vi "fourier_ring_correlation.vi"(9 "img2":dbl[][](array[numeric]), 10 "img1":dbl[][](array[numeric])) -> (1 "frc mean":dbl format="%0.2f", 2 "frc curve":dbl[][](graph))   [LabVIEW 2017]
uses:
  <vilib>/Analysis/2dsp.llb/2D Real FFT.vi
  <vilib>/Analysis/baseanly.llb/Mean (DBL).vi
  <vilib>/Analysis/3filter.llb/Zero Phase Filter (DBL).vi
  <vilib>/Analysis/NI_AALPro.lvlib
  <vilib>/Analysis/NI_AALBase.lvlib
panel:
  in  "debug":bool
  in  "power":dbl=0.1 format="%#_13g"
  out "Image":T1(plugin-control)
  in  "File Path 2":path=path "C:/Users/SiMView/Pictures/idle state-1.tif"
  in  "File Path":path=path "C:/Users/SiMView/Pictures/idle state.tif"
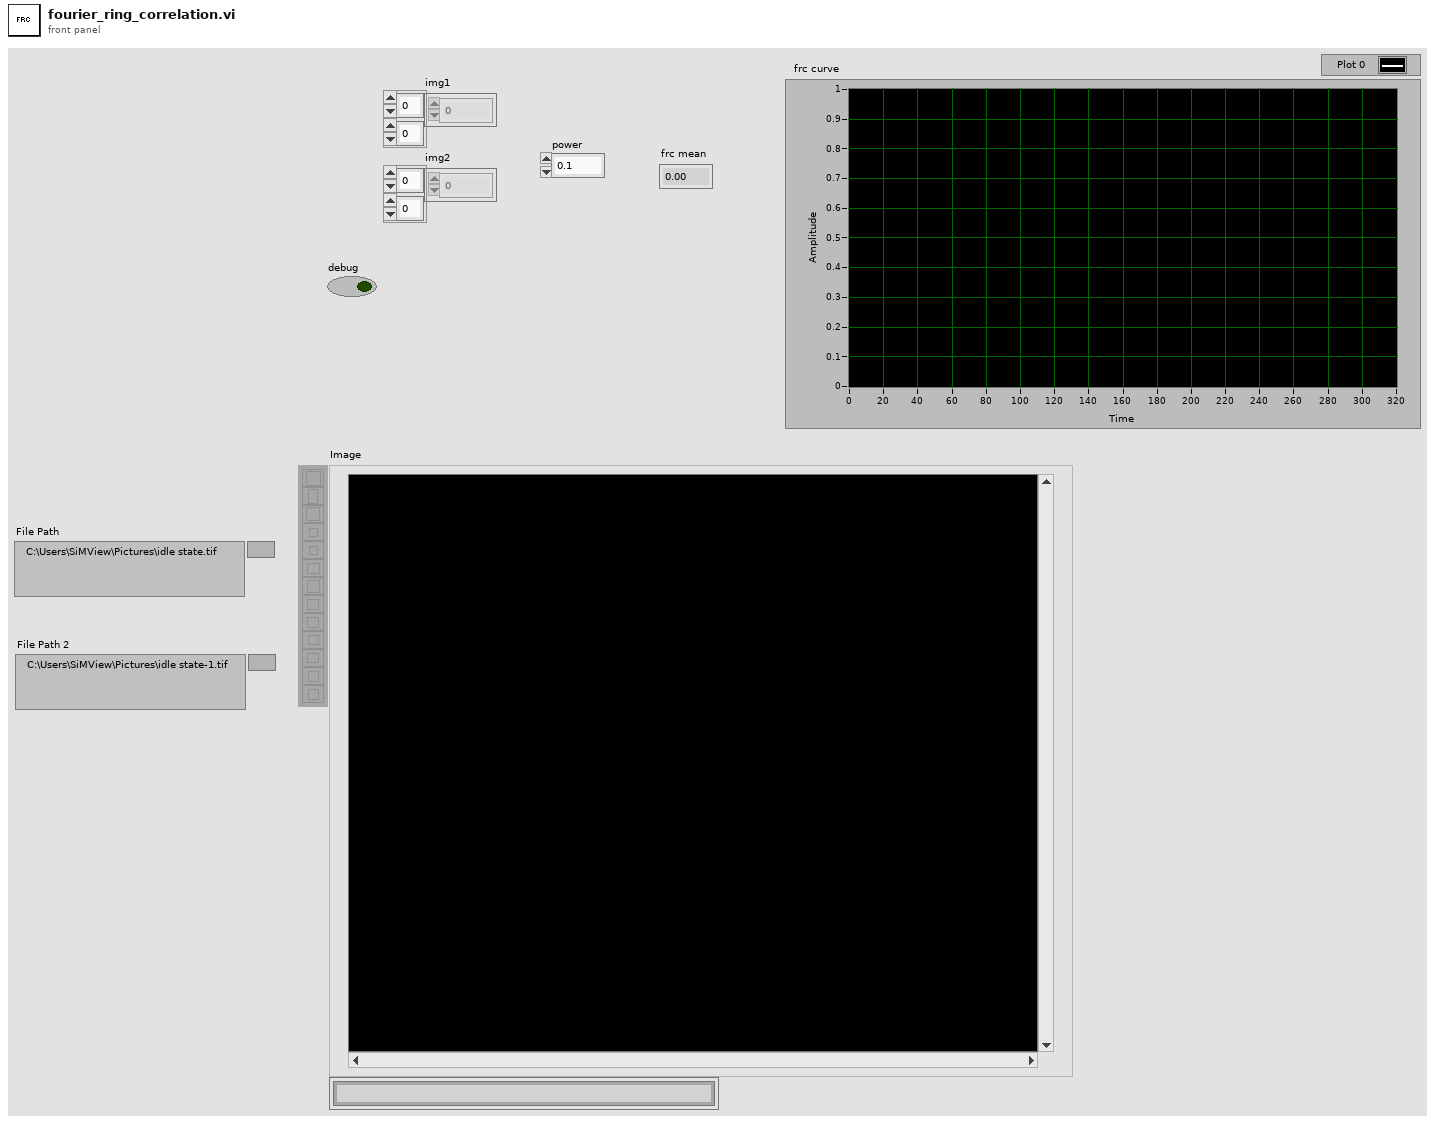
[diagram p1: front panel]
types:
  T1 = typedef "IMAQ Image.ctl" = refnum<image>
  T2 = typedef "Image Type" = u32
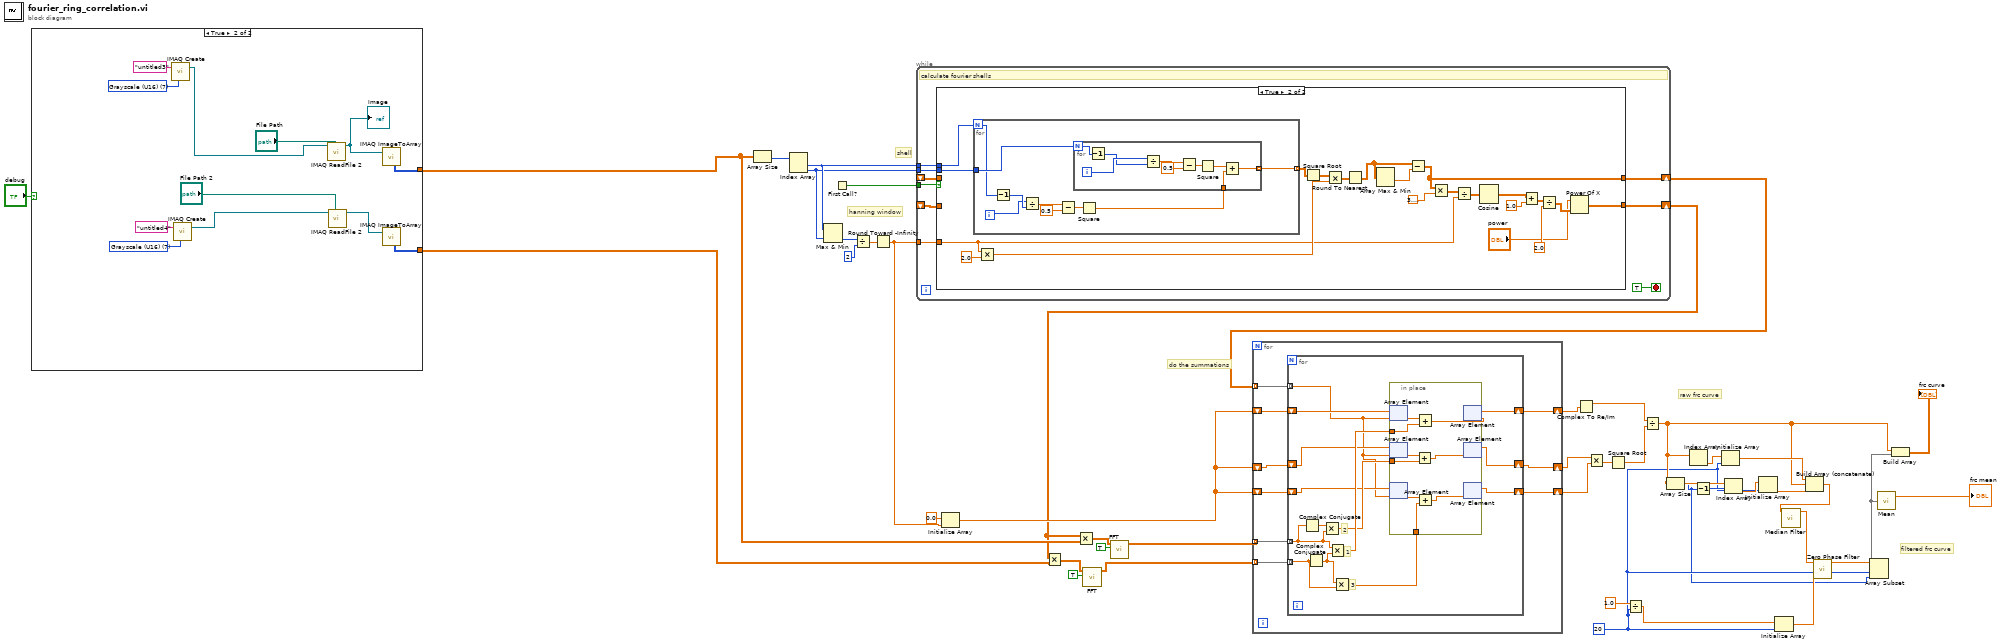
[diagram p0: block diagram]
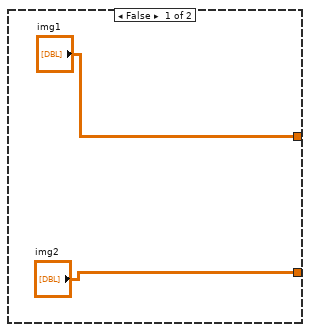
[diagram p2: hidden frame]
diagram:
  w14 = 20 ("dimension size")
  # "filtered frc curve"
  # "raw frc curve"
  # "do the summations"
  # "hanning window"
  # "shell"
  n1 = case shown="True" "debug" {
    tunnel: ["img1" w49] -> w5
    tunnel: ["img2" w47] -> w4
    frame False {
    }
    frame True {
      w53 = T2 7 items=["Grayscale (U8)", "Grayscale (I16)", "Grayscale (SGL)", "Complex (CSG)", "RGB (U32)", "HSL (U32)", "RGB (U64)", "Grayscale (U16)"] ("Image Type")
      w55 = T2 7 items=["Grayscale (U8)", "Grayscale (I16)", "Grayscale (SGL)", "Complex (CSG)", "RGB (U32)", "HSL (U32)", "RGB (U64)", "Grayscale (U16)"] ("Image Type")
      n2 = call "IMAQ Create"("Image Name"="untitled3", "Image Type"=w55) -> ("New Image"=w54:T1)  [unwired: 3 in, 1 out]
      n3 = call "IMAQ Create"("Image Name"="untitled4", "Image Type"=w53) -> ("New Image"=w51:T1)  [unwired: 3 in, 1 out]
      n4 = call "IMAQ ReadFile 2"("File Path"="File Path", "Image"=w54) -> ("Image Out"=w50:T1)  [unwired: 5 in, 4 out]
      "Image" <- w50
      n5 = call "IMAQ ReadFile 2"("File Path"="File Path 2", "Image"=w51) -> ("Image Out"=w48:T1)  [unwired: 5 in, 4 out]
      n6 = call "IMAQ ImageToArray"("Image"=w50) -> ("Image Pixels (U16)"=w49:u16[][])  [unwired: 3 in, 4 out]
      n7 = call "IMAQ ImageToArray"("Image"=w48) -> ("Image Pixels (U16)"=w47:u16[][])  [unwired: 3 in, 4 out]
    }
  }
  n8 = Array Size(array=w5) -> (size(s)=w44:i32[])
  n9 = Index Array(array=w44) -> (element #1=w40:i32, element #2=w39:i32)  [unwired: 2 in]
  n10 = Max & Min(x=w40, y=w39) -> (min(x,y)=w41:i32)  [unwired: 1 out]
  n11 = First Call?() -> (First Call?: T/F=w10:bool)
  n12 = Divide(x=w41, y=2) -> (x/y=w42:dbl)
  n13 = Round Toward -Infinity(1:w42) -> (0:w37:dbl)
  n14 = while {
    tunnel: w40 -> [w67]
    tunnel: w39 -> [w66]
    tunnel: w37 -> [w65]
    tunnel: w10 -> [w64]
    shift-right: [w61] -> w3
    shift-left: _ -> [w62]
    shift-right: [w59] -> w2
    shift-left: _ -> [w60]
    stop <- TRUE stop-if-true
    # "calculate fourier shells"
    n15 = case shown="True" w64 {
      tunnel: w67 -> [_ w90]
      tunnel: w66 -> [_ w89]
      tunnel: w65 -> [_ w78]
      tunnel: w62 -> [w69 _]
      tunnel: [w69 w81] -> w61
      tunnel: w60 -> [w68 _]
      tunnel: [w68 w72] -> w59
      frame False {
      }
      frame True {
        n16 = for {
          N: w90 -> [w95]
          tunnel: w89 -> [w99]
          tunnel: [w91] -> w86 mode=indexing
          i -> [w94]
          n17 = Decrement(x=w95) -> (x-1=w96:i32)
          n18 = Divide(x=w94, y=w96) -> (x/y=w97:dbl)
          n19 = Subtract(x=w97, y=0.5) -> (x-y=w93:dbl)
          n20 = Square(x=w93) -> (x^2=w92:dbl)
          n21 = for {
            N: w99 -> [w107]
            tunnel: w92 -> [w101]
            tunnel: [w100] -> w91 mode=indexing
            i -> [w108]
            n22 = Decrement(x=w107) -> (x-1=w106:i32)
            n23 = Divide(x=w108, y=w106) -> (x/y=w105:dbl)
            n24 = Subtract(x=w105, y=0.5) -> (x-y=w103:dbl)
            n25 = Square(x=w103) -> (x^2=w102:dbl)
            n26 = Add(x=w102, y=w101) -> (x+y=w100:dbl)
          }
        }
        n27 = Multiply(x=w78, y=2.0) -> (x*y=w84:dbl)
        n28 = Square Root(x=w86) -> (sqrt(x)=w87:dbl[][])
        n29 = Multiply(x=w87, y=w84) -> (x*y=w88:dbl[][])
        n30 = Round To Nearest(number=w88) -> (nearest integer value=w82:dbl[][])
        n31 = Array Max & Min(array=w82) -> (min value=w83:dbl)  [unwired: 3 out]
        n32 = Subtract(x=w82, y=w83) -> (x-y=w81:dbl[][])
        n33 = Multiply(x=w81, y=3.141592653589793) -> (x*y=w79:dbl[][])
        n34 = Divide(x=w79, y=w78) -> (x/y=w77:dbl[][])
        n35 = Cosine(x=w77) -> (cos(x)=w76:dbl[][])
        n36 = Add(x=w76, y=1.0) -> (x+y=w74:dbl[][])
        n37 = Divide(x=w74, y=2.0) -> (x/y=w71:dbl[][])
        n38 = Power Of X(1:w71, 2:"power") -> (0:w72:dbl[][])
      }
    }
  }
  n39 = Initialize Array(0.0 ("element"), w37) -> (w36:dbl[])
  n40 = Multiply(x=w2, y=w4) -> (x*y=w9:dbl[][])
  n41 = Multiply(x=w2, y=w5) -> (x*y=w7:dbl[][])
  n42 = call-poly <vilib>:"FFT.vi"("shift?"=TRUE, "X"=w9) -> ("FFT {X}"=w8:cdb[][])  [unwired: 8 in, 1 out]
  n43 = call-poly <vilib>:"FFT.vi"("shift?"=TRUE, "X"=w7) -> ("FFT {X}"=w6:cdb[][])  [unwired: 8 in, 1 out]
  n44 = for {
    tunnel: w6 -> [w111] mode=indexing
    tunnel: w8 -> [w110] mode=indexing
    tunnel: w3 -> [w109] mode=indexing
    shift-right: [w114] -> w32
    shift-left: w36 -> [w117]
    shift-right: [w113] -> w35
    shift-left: w36 -> [w116]
    shift-right: [w112] -> w34
    shift-left: w36 -> [w115]
    n45 = for {
      tunnel: w109 -> [w120] mode=indexing
      tunnel: w111 -> [w130] mode=indexing
      tunnel: w110 -> [w128] mode=indexing
      shift-right: [w125] -> w114
      shift-left: w117 -> [w127]
      shift-right: [w122] -> w113
      shift-left: w116 -> [w124]
      shift-right: [w118] -> w112
      shift-left: w115 -> [w121]
      # "3"
      # "2"
      # "1"
      n46 = Complex Conjugate(1:w130) -> (0:w131:cdb)
      n47 = Complex Conjugate(1:w128) -> (0:w129:cdb)
      n48 = Multiply(x=w131, y=w130) -> (x*y=w123:cdb)
      n49 = Multiply(x=w130, y=w129) -> (x*y=w126:cdb)
      n50 = Multiply(x=w129, y=w128) -> (x*y=w119:cdb)
      n51 = in-place {
        in-place-border: w126 -> [w139]
        in-place-border: w123 -> [w136]
        in-place-border: w119 -> [w133]
        n52 = in-place-array #1(w127, w120) -> (w140:dbl)
        n53 = in-place-array #2(w124, w120) -> (w137:dbl)
        n54 = in-place-array #3(w121, w120) -> (w134:dbl)
        n55 = Add(x=w137, y=w136) -> (x+y=w135:cdb)
        n56 = Add(x=w140, y=w139) -> (x+y=w138:cdb)
        n57 = Add(x=w134, y=w133) -> (x+y=w132:cdb)
        n58 = in-place-array #1(w138) -> (w125:dbl[])  [unwired: 1 out]
        n59 = in-place-array #2(w135) -> (w122:dbl[])  [unwired: 1 out]
        n60 = in-place-array #3(w132) -> (w118:dbl[])  [unwired: 1 out]
      }
    }
  }
  n61 = Complex To Re/Im(x + iy=w32) -> (x=w31:dbl[])  [unwired: 1 out]
  n62 = Multiply(x=w35, y=w34) -> (x*y=w33:dbl[])
  n63 = Square Root(x=w33) -> (sqrt(x)=w30:dbl[])
  n64 = Divide(x=1.0 ("element"), y=w14) -> (x/y=w23:dbl)
  n65 = Divide(x=w31, y=w30) -> (x/y=w19:dbl[])
  n66 = Array Size(array=w19) -> (size(s)=w13:i32)
  n67 = Index Array(array=w19) -> (element=w22:dbl)  [unwired: 1 in]
  n68 = Decrement(x=w13) -> (x-1=w20:i32)
  n69 = Initialize Array(w22, w14) -> (w21:dbl[])
  n70 = Index Array(array=w19, index=w20) -> (element=w18:dbl)
  n71 = Initialize Array(w18, w14) -> (w17:dbl[])
  n72 = Initialize Array(w23, w14) -> (w27:dbl[])
  n73 = Build Array (concatenate)(w21, w19, w17) -> (w16:dbl[])
  n74 = call <vilib>:"Median Filter.vi"("X"=w16) -> ("Filtered X"=w25:dbl[])  [unwired: 9 in, 1 out]
  n75 = call-poly <vilib>:"Zero Phase Filter.vi"("Forward Coefficients"=w27, "X"=w25) -> ("Filtered X"=w15:dbl[])  [unwired: 8 in, 1 out]
  n76 = Array Subset(array=w15, index=w14, length=w13) -> (w12:dbl[])
  n77 = call-poly <vilib>:"Mean.vi"("X"=w12) -> ("mean"=→"frc mean":dbl)  [unwired: 1 out]
  n78 = Build Array(w19, w12) -> (→"frc curve":dbl[][])
